vi "Merge images.vi"(0 "Image types":u32[](array[numeric]), 1 "ROI":i32[](array[numeric])=[0, 0, 32767, 32767], 2 "File paths":path[](array[path]), 3 "RGB image buffers in":T1[](array[typedef]), 5 "Overlay frame numbers":u32[](array[numeric]), 7 "Black/white levels":cluster{ext, ext}[](array[cluster]), 9 "8 bit scratch images":T1[](array[typedef]), 10 "Write text overlay?":bool, 11 "error in":errorcluster, 12 "N-bit images in":T1[](array[typedef]), 13 "Transform types":string[](array[string]), 14 "Transform number?":u16, 15 "Image colors":u32[](array[numeric])) -> (4 "N-bit images out":T1[](array[typedef]), 6 "RGB Image out":T1, 8 "error out":errorcluster)   [LabVIEW 2011]
doc: "Makes a pseudo-color aligned merged image from two monochrome images collected at different wavelengths."
uses:
  <vilib>/vision/Image Controls.llb/IMAQ Image.ctl
  <vilib>/vision/NI_Vision_Development_Module.lvlib
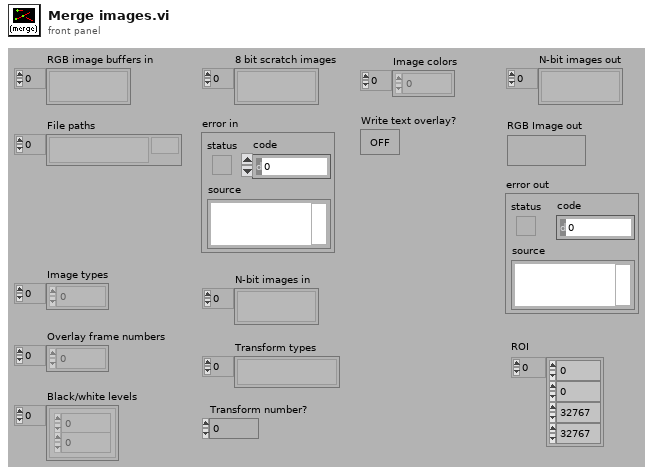
[diagram p1: front panel]
types:
  T1 = typedef "IMAQ Image.ctl" = refnum<image>
  T2 = cluster{"Red (or Hue) value":u8, "Green (or Sat) value":u8, "Blue (or Light or Val) value":u8}
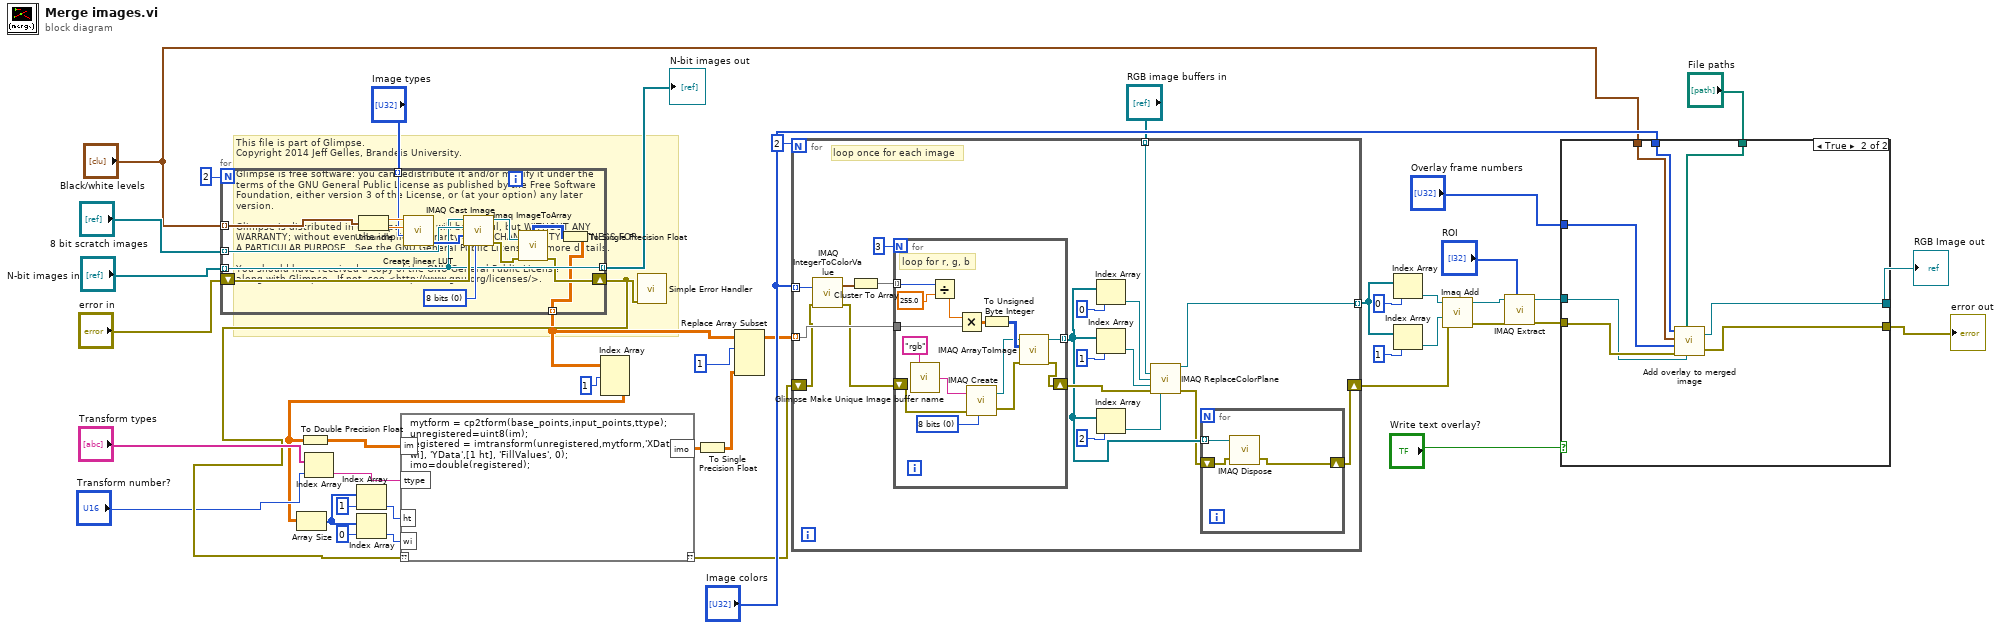
[diagram p0: block diagram]
diagram:
  # "This file is part of Glimpse. \nCopyright 2014 Jeff Gelles, Brandeis University.    \n\nGlimpse is free software: you can redistribute it and/or modify it under the \nterms of the GNU General Public License as published by the Free Software \nFoundation, either version 3 of the License, or (at your option) any later \nversion.\n\nGlimpse is distributed in the hope that it will be useful, but WITHOUT ANY \nWARRANTY; without even the implied warranty of MERCHANTABILITY or FITNESS FOR \nA PARTICULAR PURPOSE.  See the GNU General Public License for more details.\n\nYou should have received a copy of the GNU General Public License\nalong with Glimpse.  If not, see <http://www.gnu.org/licenses/>."
  n1 = for {
    N: 2 -> [_]
    shift-right: [w49] -> w43
    shift-left: "error in" -> [w54]
    tunnel: [w52] -> w30 mode=indexing
    tunnel: "8 bit scratch images" -> [w55] mode=indexing
    tunnel: "N-bit images in" -> [w52] mode=indexing
    tunnel: [w47] -> w19 mode=indexing
    tunnel: "Image types" -> [w46] mode=indexing
    tunnel: "Black/white levels" -> [w45] mode=indexing
    w53 = u32 0 items=["8 bits", "16 bits", "Float", "Complex", "RGB", "HSL"] ("Image Type")
    n2 = Unbundle(w45) -> (w58:ext, w57:ext)
    n3 = call "Create linear LUT.vi"("Input Image Type"=w46, "White Value"=w57, "Black Value"=w58) -> ("LUT (U8) Out"=w56:u8[])  [unwired: 6 out]
    n4 = call "IMAQ Cast Image"("Image Type"=w53, "error in (no error)"=w54, "Lookup Table"=w56, "Image Dst"=w55, "Image Src"=w52) -> ("error out"=w50:errorcluster, "Image Dst Out"=w51:T1)  [unwired: 1 in, 4 out]
    n5 = call "Imaq ImageToArray"("error in (no error)"=w50, "Image"=w51) -> ("error out"=w49:errorcluster, "Image Pixels (U8)"=w48:u8[][])  [unwired: 1 in, 4 out]
    n6 = To Single Precision Float(number=w48) -> (single precision float=w47:sgl[][])
  }
  "N-bit images out" <- w30
  n7 = Index Array(array="Transform types", index="Transform number?") -> (element=w11:string)
  n8 = Index Array(array=w19, index (dim 0)=1 ("disabled index (col)")) -> (element=w17:sgl[][])  [unwired: 2 in]
  n9 = Array Size(array=w17) -> (size(s)=w16:i32[])
  n10 = To Double Precision Float(number=w17) -> (double precision float=w10:dbl[][])
  n11 = Index Array(array=w16, index=1) -> (element=w14:i32)
  n12 = Index Array(array=w16, index=0) -> (element=w15:i32)
  n13 = script code="mytform = cp2tform(base_points,input_points,ttype);\nunregistered=uint8(im);\nregistered = imtransform(unregistered,mytform,'XData',[1 wi], 'YData',[1 ht], 'FillValues', 0);\nimo=double(registered);"("??"=w43, "im"=w10, "ht"=w14, "wi"=w15, "ttype"=w11) -> ("??"=w23:errorcluster, "imo"=w18:dbl[][])
  n14 = call <vilib>:"Simple Error Handler.vi"("error in (no error)"=w43) -> ()  [unwired: 1 in, 8 out]
  n15 = To Single Precision Float(number=w18) -> (single precision float=w20:sgl[][])
  n16 = Replace Array Subset(array=w19, new element=w20, index (dim 0)=1 ("disabled index (col)")) -> (w21:sgl[][][])  [unwired: 2 in]
  n17 = for {
    N: 2 -> [_]
    tunnel: "Image colors" -> [w77] mode=indexing
    tunnel: w21 -> [w74] mode=indexing
    shift-right: [w60] -> w34
    shift-left: w23 -> [w72]
    tunnel: "RGB image buffers in" -> [w62] mode=indexing
    tunnel: [w63] -> w27 mode=indexing
    # "loop once for each image"
    n18 = call "IMAQ IntegerToColorValue"("error in (no error)"=w72, "U32 value"=w77) -> ("error out"=w71:errorcluster, "Color Value"=w76:T2)  [unwired: 3 in, 2 out]
    n19 = Cluster To Array(cluster=w76) -> (array=w75:u8[])
    n20 = for {
      N: 3 -> [_]
      tunnel: w75 -> [w93] mode=indexing
      tunnel: w74 -> [w91]
      tunnel: [w83] -> w61 mode=indexing
      shift-right: [w81] -> w65
      shift-left: w71 -> [w82]
      w87 = u32 0 items=["8 bits", "16 bits", "Float", "Complex", "RGB", "HSL"] ("Image Type")
      # "loop for r, g, b"
      n21 = call "Glimpse Make Unique Image buffer name.vi"("Buffer  base name"="rgb") -> ("Image Name"=w89:string)  [unwired: 1 out]
      n22 = Divide(x=w93, y=255.0) -> (x/y=w92:dbl)
      n23 = Multiply(x=w92, y=w91) -> (x*y=w90:dbl[][])
      n24 = call "IMAQ Create"("Image Name"=w89, "Image Type"=w87, "error in (no error)"=w82) -> ("New Image"=w85:T1, "error out"=w84:errorcluster)  [unwired: 1 in, 1 out]
      n25 = To Unsigned Byte Integer(number=w90) -> (unsigned 8bit integer=w86:u8[][])
      n26 = call "IMAQ ArrayToImage"("error in (no error)"=w84, "Image Pixels (U8)"=w86, "Image"=w85) -> ("error out"=w81:errorcluster, "Image Out"=w83:T1)  [unwired: 3 in, 4 out]
    }
    n27 = Index Array(array=w61, index=0 ("disabled index (col)")) -> (element=w66:T1)
    n28 = Index Array(array=w61, index=1 ("disabled index (col)")) -> (element=w67:T1)
    n29 = Index Array(array=w61, index=2 ("disabled index (col)")) -> (element=w64:T1)
    n30 = call "IMAQ ReplaceColorPlane"("Image Dst"=w62, "Red or Hue Plane"=w66, "Green or Sat Plane"=w67, "error in (no error)"=w65, "Blue or Luma or Val or Inten Plane"=w64) -> ("Image Dst Out"=w63:T1, "error out"=w59:errorcluster)  [unwired: 2 in, 7 out]
    n31 = for {
      tunnel: w61 -> [w80] mode=indexing
      shift-right: [w78] -> w60
      shift-left: w59 -> [w79]
      n32 = call "IMAQ Dispose"("Image"=w80, "error in (no error)"=w79) -> ("error out"=w78:errorcluster)  [unwired: 1 in, 3 out]
    }
  }
  n33 = Index Array(array=w27, index=0 ("disabled index (col)")) -> (element=w28:T1)
  n34 = Index Array(array=w27, index=1 ("disabled index (col)")) -> (element=w29:T1)
  n35 = call "Imaq Add"("Image Src A"=w28, "Image Src B"=w29, "error in (no error)"=w34) -> ("Image Dst Out"=w3:T1, "error out"=w5:errorcluster)  [unwired: 2 in, 2 out]
  n36 = call "IMAQ Extract"("Optional Rectangle"="ROI", "error in (no error)"=w5, "Image Src"=w3) -> ("error out"=w4:errorcluster, "Image Dst Out"=w2:T1)  [unwired: 3 in, 4 out]
  n37 = case shown="True" "Write text overlay?" {
    tunnel: "Image colors" -> [_ w104]
    tunnel: w4 -> [w95 w103]
    tunnel: [w95 w99] -> w40
    tunnel: w2 -> [w96 w102]
    tunnel: [w96 w98] -> w41
    tunnel: "File paths" -> [_ w101]
    tunnel: "Black/white levels" -> [_ w100]
    tunnel: "Overlay frame numbers" -> [_ w97]
    frame False {
    }
    frame True {
      n38 = call "Add overlay to merged image.vi"("Image in"=w102, "File paths"=w101, "error in"=w103, "Overlay frame numbers"=w97, "Black/White levels"=w100, "Overlay colors"=w104) -> ("error out"=w99:errorcluster, "Image Out"=w98:T1)
    }
  }
  "RGB Image out" <- w41
  "error out" <- w40
